vi "Read Page.vi"(7 "index":i32, 8 "error in (no error)":errorcluster, 9 "Page Info":T4(array[cluster]), 10 "Tiff Bitness":T5(ring), 11 "Byte Stream File in":refnum<file>) -> (0 "error out":errorcluster, 1 "Details":T3={"ImageDescription"="", "XResolution"=0.0, "YResolution"=0.0, "ResolutionUnit"=enum."Inch", "PhotometricInterpretation"=0, "Compression"=enum."None", "PageName"="", "DocumentName"=""} {"PhotometricInterpretation" items=["PHOTOMETRIC_MINISWHITE"=0, "PHOTOMETRIC_MINISBLACK"=1, "PHOTOMETRIC_RGB"=2, "PHOTOMETRIC_PALETTE"=3, "PHOTOMETRIC_MASK"=4, "PHOTOMETRIC_SEPARATED"=5, "PHOTOMETRIC_YCBCR"=6, "PHOTOMETRIC_CIELAB"=8, "PHOTOMETRIC_ICCLAB"=9, "PHOTOMETRIC_ITULAB"=10, "PHOTOMETRIC_LOGL"=32844, "PHOTOMETRIC_LOGLUV"=32845, "CFA"=32803, "LinearRaw"=34892, "DEPTH"=51177]}, 2 "Variant":variant, 3 "Byte Stream File out":refnum<file>, 4 "IFD Info":T2(c390))   [LabVIEW 2020, in "LV Tiff.lvlib"]
uses:
  LV Tiff.lvlib
  Tiff Data Type.ctl
  Tiff Page Details.ctl
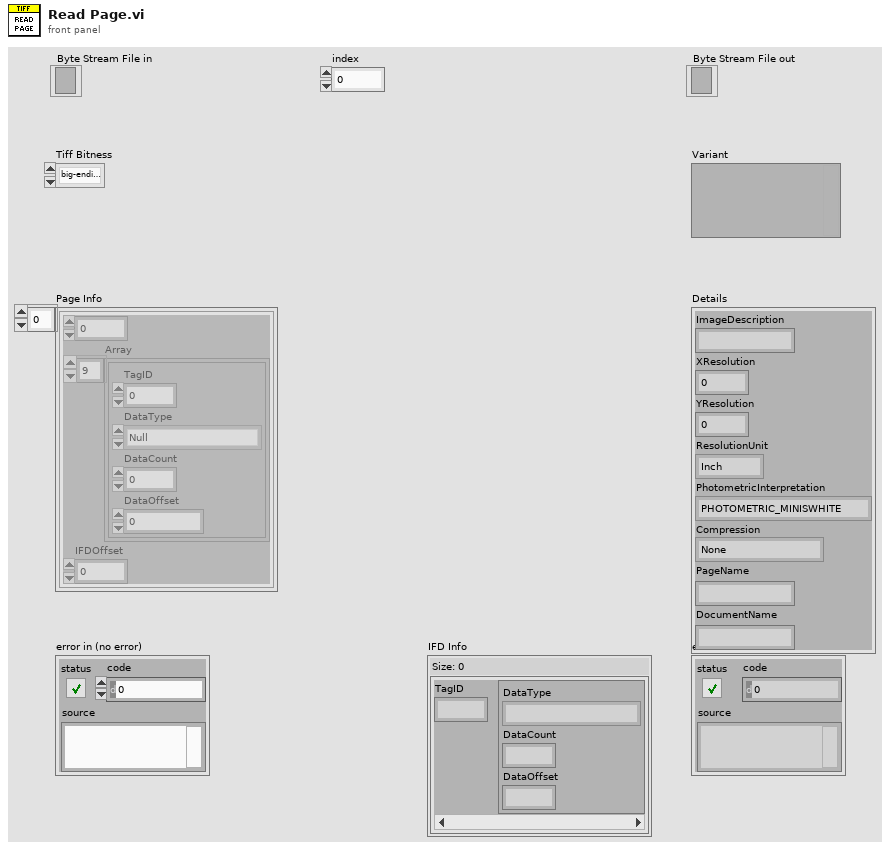
[diagram p1: front panel]
types:
  T1 = typedef "LV Tiff.lvlib/Tiff Data Type.ctl" = enum16{"Null", "BYTE", "ASCII", "SHORT", "LONG", "RATIONAL", "SBYTE", "UNDEFINE", "SSHORT", "SLONG", "SRATIONAL", "FLOAT", "DOUBLE"}
  T2 = map{u16, cluster{"DataType":T1, "DataCount":u32, "DataOffset":u32}}
  T3 = typedef "LV Tiff.lvlib/Tiff Page Details.ctl" = cluster{"ImageDescription":string, "XResolution":dbl, "YResolution":dbl, "ResolutionUnit":enum16{"None", "Inch", "Centimeter"}, "PhotometricInterpretation":u16, "Compression":enum16{"None", "Deflate"}, "PageName":string, "DocumentName":string}
  T4 = cluster{i32, "Array":cluster{"TagID":u16, "DataType":T1, "DataCount":u32, "DataOffset":u32}[], "IFDOffset":u32}[]
  T5 = enum16{"big-endian, network order", "native, host order", "little-endian"}
  T6 = cluster{i32, "Array":cluster{"TagID":u16, "DataType":T1, "DataCount":u32, "DataOffset":u32}[], "IFDOffset":u32}
  T7 = typedef "LV Tiff.lvlib/Baseline Tags 1.ctl" = cluster{"NewSubFileType":u32, "ImageWidth":u32, "ImageHeight":u32, "BitsPerSample":u16, "Compression":u16, "PhotometricInterpretation":u16, "StripOffsets":u32[], "SamplesPerPixel":u16, "RowsPerStrip":u32, "StripByteCounts":u32[], "ResolutionUnit":u16, "SampleFormat":u16}
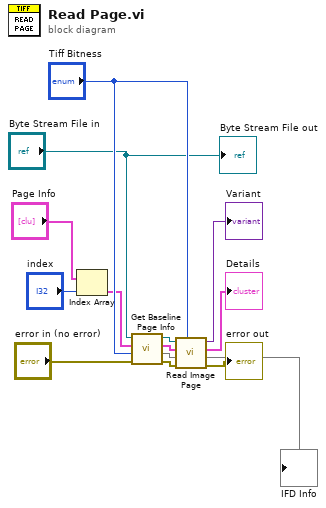
[diagram p0: block diagram]
diagram:
  n1 = Index Array(array="Page Info", index="index") -> (element=w5:T6)
  n2 = call "Get Baseline Page Info.vi"("error in 2"="error in (no error)", "Tiff Bitness"="Tiff Bitness", "Page Info"=w5, "Byte Stream File in"="Byte Stream File in") -> ("error out"=w12:errorcluster, "IFDO Info"=w1:T2, "Page Info"=w6:T7, "Byte Stream File out"=w7:refnum<file>)  [unwired: 4 in]
  "IFD Info" <- w1
  n3 = call "Read Image Page.vi"("Tiff Bitness"="Tiff Bitness", "error in (no error)"=w12, "IFDO Info"=w1, "Page Info"=w6, "Byte Stream File in"=w7) -> ("error out"=→"error out":errorcluster, "Details"=→"Details":T3, "Variant Strips"=→"Variant":variant)  [unwired: 4 in]
  "Byte Stream File out" <- "Byte Stream File in"
